vi "Config Type.vi"(11 "Error Command in":refnum<class "Error Command.lvclass">) -> (2 "Command Config Type":refnum<class "Command Config.lvclass">)   [LabVIEW 2020, in "VolatusSeq.lvlib" / "Error Command.lvclass"]
uses:
  Error Command.lvclass
  Error Command.lvclass/Error Command.ctl
  VolatusSeqConfig/Error Command Config/Error Command Config.lvclass
  C:/dev/lv20CE/relink/lv-volatus/VolatusSeqConfig/Command Config/Command Config.lvclass
  C:/dev/lv20CE/relink/lv-volatus/VolatusSeqConfig/Error Command Config/Error Command Config.lvclass
  VolatusSeqConfig/Command Config/Command Config.lvclass
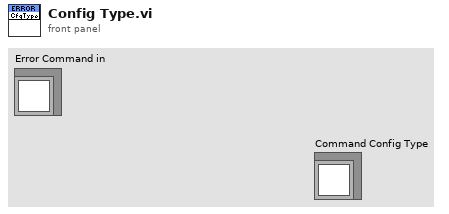
[diagram p1: front panel]
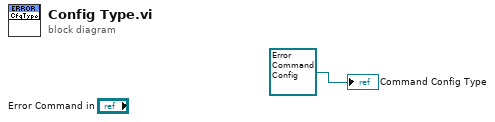
[diagram p0: block diagram]
diagram:
  "Command Config Type" <- refnum<class "Error Command Config.lvclass"> refnum ("VolatusSeqConfig.lvlib:Error Command Config.lvclass")
